vi "save image.vi"(1 "Start of pump/prove run?":bool, 2 "Image to save":i32[][](array[numeric]), 3 "Pump/probe run?":bool) -> (0 "Image file path":string)   [LabVIEW 2019]
uses:
  <vilib>/Utility/file.llb/Write Delimited Spreadsheet (I64).vi
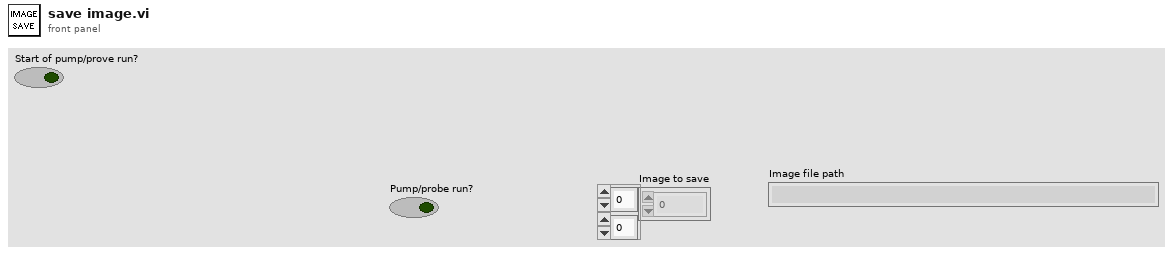
[diagram p1: front panel]
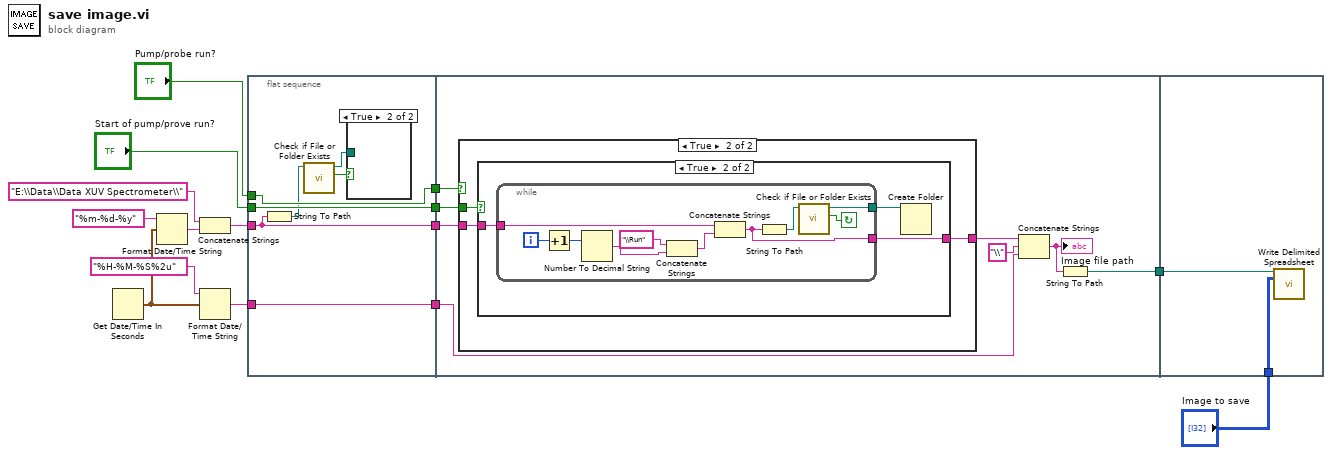
[diagram p0: block diagram]
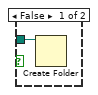
[diagram p2: hidden frame]
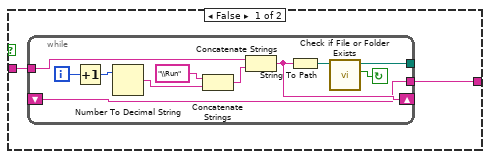
[diagram p4: hidden frame]
diagram:
  n1 = Get Date/Time In Seconds() -> (seconds since 1Jan1904=w14:timestamp)
  n2 = Format Date/Time String(time format string (%c)="%m-%d-%y", seconds (now)=w14) -> (date/time string=w15:string)  [unwired: 1 in]
  n3 = Concatenate Strings("E:\\Data\\Data XUV Spectrometer\\" ("string"), w15) -> (w9:string)
  n4 = Format Date/Time String(time format string (%c)="%H-%M-%S%2u", seconds (now)=w14) -> (date/time string=w8:string)  [unwired: 1 in]
  n5 = flat-sequence {
    tunnel: "Start of pump/prove run?" -> [w19]
    tunnel: "Pump/probe run?" -> [w20]
    tunnel: w8 -> [w21]
    tunnel: w9 -> [w22]
    tunnel: [w22] -> w4
    tunnel: [w21] -> w3
    tunnel: [w20] -> w2
    tunnel: [w19] -> w1
    tunnel: [w28] -> w7
    tunnel: w4 -> [w24]
    tunnel: w3 -> [w29]
    tunnel: w2 -> [w26]
    tunnel: w1 -> [w25]
    tunnel: "Image to save" -> [w63]
    tunnel: w7 -> [w62]
    frame #0 {
      n6 = String To Path(string=w22) -> (path=w18:path)
      n7 = call <vilib>:"Check if File or Folder Exists.vi"("path"=w18) -> ("file or folder exists?"=w17:bool, "dup path"=w16:path)  [unwired: 8 in, 1 out]
      n8 = case shown="True" w17 {
        tunnel: w16 -> [w23 _]
        frame False {
          n9 = Create Folder(path (use dialog)=w23) -> ()  [unwired: 2 in, 3 out]
        }
        frame True {
        }
      }
    }
    frame #1 {
      n10 = case shown="True" w26 {
        tunnel: w24 -> [w32 w35]
        tunnel: [w32 w34] -> w27
        tunnel: w25 -> [_ w33]
        frame False {
        }
        frame True {
          n11 = case shown="True" w33 {
            tunnel: w35 -> [w37 w51]
            tunnel: [w36 w49] -> w34
            frame False {
              n12 = while {
                tunnel: w37 -> [w47]
                tunnel: [w42] -> _
                shift-right: [w41] -> _
                shift-left: _ -> [w38]
                tunnel: [w38] -> w36
                i -> [w40]
                stop <- w43 continue-if-true
                n13 = Increment(x=w40) -> (x+1=w39:i32)
                n14 = Number To Decimal String(number=w39) -> (decimal integer string=w44:string)  [unwired: 1 in]
                n15 = Concatenate Strings("\\Run" ("string"), w44) -> (w46:string)
                n16 = Concatenate Strings(w47, w46) -> (w41:string)
                n17 = String To Path(string=w41) -> (path=w45:path)
                n18 = call <vilib>:"Check if File or Folder Exists.vi"("path"=w45) -> ("file or folder exists?"=w43:bool, "dup path"=w42:path)  [unwired: 8 in, 1 out]
              }
            }
            frame True {
              n19 = while {
                tunnel: w51 -> [w60]
                tunnel: [w55] -> w50
                tunnel: [w54] -> w49
                i -> [w53]
                stop <- w56 continue-if-true
                n20 = Increment(x=w53) -> (x+1=w52:i32)
                n21 = Number To Decimal String(number=w52) -> (decimal integer string=w57:string)  [unwired: 1 in]
                n22 = Concatenate Strings("\\Run" ("string"), w57) -> (w59:string)
                n23 = Concatenate Strings(w60, w59) -> (w54:string)
                n24 = String To Path(string=w54) -> (path=w58:path)
                n25 = call <vilib>:"Check if File or Folder Exists.vi"("path"=w58) -> ("file or folder exists?"=w56:bool, "dup path"=w55:path)  [unwired: 8 in, 1 out]
              }
              n26 = Create Folder(path (use dialog)=w50) -> ()  [unwired: 2 in, 3 out]
            }
          }
        }
      }
      n27 = Concatenate Strings(w27, "\\" ("string"), w29) -> (w31:string)
      "Image file path" <- w31
      n28 = String To Path(string=w31) -> (path=w28:path)
    }
    frame #2 {
      n29 = call-poly <vilib>:"Write Delimited Spreadsheet.vi"("file path (dialog if empty)"=w62, "2D data"=w63) -> ()  [unwired: 12 in, 2 out]
    }
  }
